vi "Write Single Channel Setting.vi"(8 "error in (no error)":errorcluster, 9 "Channel Setting":T1={"Amplitude"=0.0, "Vertical Coupling"=enum."DC", "Probe Attenuation"=0.0, "Enable?"=FALSE, "Maximum Input Frequency"=0.0, "Input Impedance"=0, "Timeout (s)"=5.0} {"Timeout (s)" format="%.2f"; "Input Impedance" items=["1 mega ohm", "50 ohms"]; "Maximum Input Frequency" format="%.2f"}, 10 "Channel List":T3 items=["Channel_1", "Channel_2", "Channel_3", "Channel_4", "Channel_5", "Channel_6", "Channel_7", "Channel_8"], 11 "Oscilloscope in":refnum<class "Oscilloscope.lvclass">) -> (0 "error out":errorcluster, 3 "Oscilloscope out":refnum<class "Oscilloscope.lvclass">)   [LabVIEW 2019, in "Oscilloscope.lvlib" / "Oscilloscope.lvclass"]
uses:
  Oscilloscope.lvclass
  Custom Controls/Channel List.ctl
  Custom Controls/Channel Settings.ctl
  Custom Controls/Vertical Coupling.ctl
  Oscilloscope.lvclass/Oscilloscope.ctl
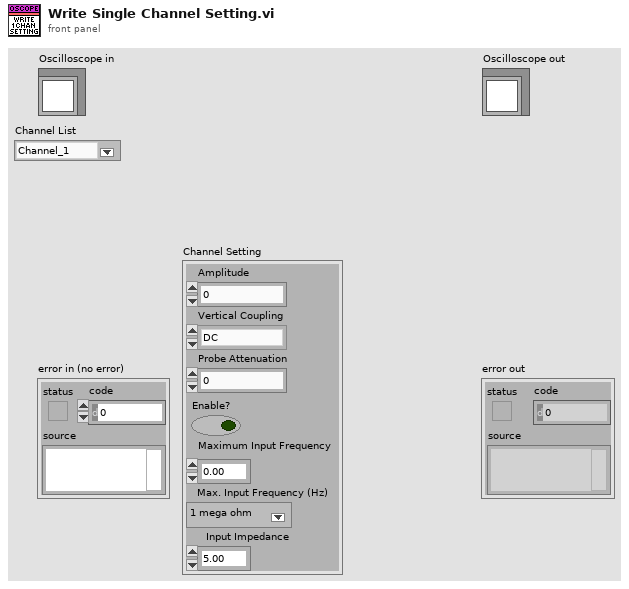
[diagram p1: front panel]
types:
  T1 = typedef "Oscilloscope.lvlib/Oscilloscope.lvclass/Channel Settings.ctl" = cluster{"Amplitude":dbl, "Vertical Coupling":T2, "Probe Attenuation":dbl, "Enable?":bool, "Maximum Input Frequency":dbl, "Input Impedance":u16, "Timeout (s)":dbl}
  T2 = typedef "Oscilloscope.lvlib/Oscilloscope.lvclass/Vertical Coupling.ctl" = enum16{"AC", "DC", "Ground"}
  T3 = typedef "Oscilloscope.lvlib/Oscilloscope.lvclass/Channel List.ctl" = u16
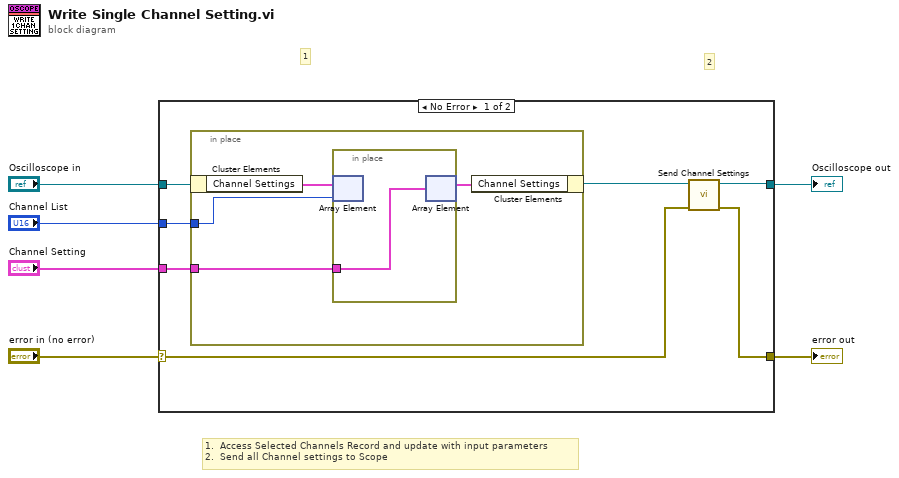
[diagram p0: block diagram]
diagram:
  # "1.  Access Selected Channels Record and update with input parameters\n2.  Send all Channel settings to Scope"
  # "2"
  # "1"
  n1 = case shown="No Error" "error in (no error)" {
    selector: "error in (no error)" -> [w8 w20]
    tunnel: "Oscilloscope in" -> [w13 w19]
    tunnel: [w11 w19] -> w5
    tunnel: "Channel List" -> [w10 _]
    tunnel: "Channel Setting" -> [w9 _]
    tunnel: [w7 w20] -> w1
    frame No Error {
      n2 = in-place {
        in-place-border: w10 -> [w15]
        in-place-border: w9 -> [w14]
        n3 = in-place-cluster #1(w13) -> ("Channel Settings"=w17:T1[])
        n4 = in-place {
          in-place-border: w14 -> [w18]
          n5 = in-place-array #2(w17, w15) -> ()  [unwired: 1 out]
          n6 = in-place-array #2(w18) -> (w16:T1[])  [unwired: 1 out]
        }
        n7 = in-place-cluster #1("Channel Settings"=w16) -> (w12:refnum<class "Oscilloscope.lvclass">)
      }
      n8 = call-dynamic "Send Channel Settings.vi"("error in (no error)"=w8, "Oscilloscope in"=w12) -> ("error out"=w7:errorcluster, "Oscilloscope out"=w11:refnum<class "Oscilloscope.lvclass">)  [unwired: 8 in]
    }
    frame Error {
    }
  }
  "error out" <- w1
  "Oscilloscope out" <- w5
